vi "DS18S20 - read temp.vi"() -> ()   [LabVIEW 2012]
panel:
  out "Loop Rate (tics)":u32
  in  "stop":bool
  out "Scratchpad Data":u8[](array[numeric]) format="%.0x"
  out "ROM Data":u8[](array[numeric]) format="%.0x"
  out "error out":errorcluster
  in  "error in":errorcluster
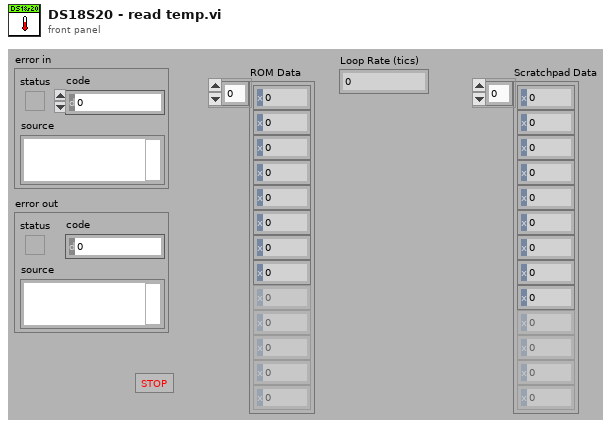
[diagram p1: front panel]
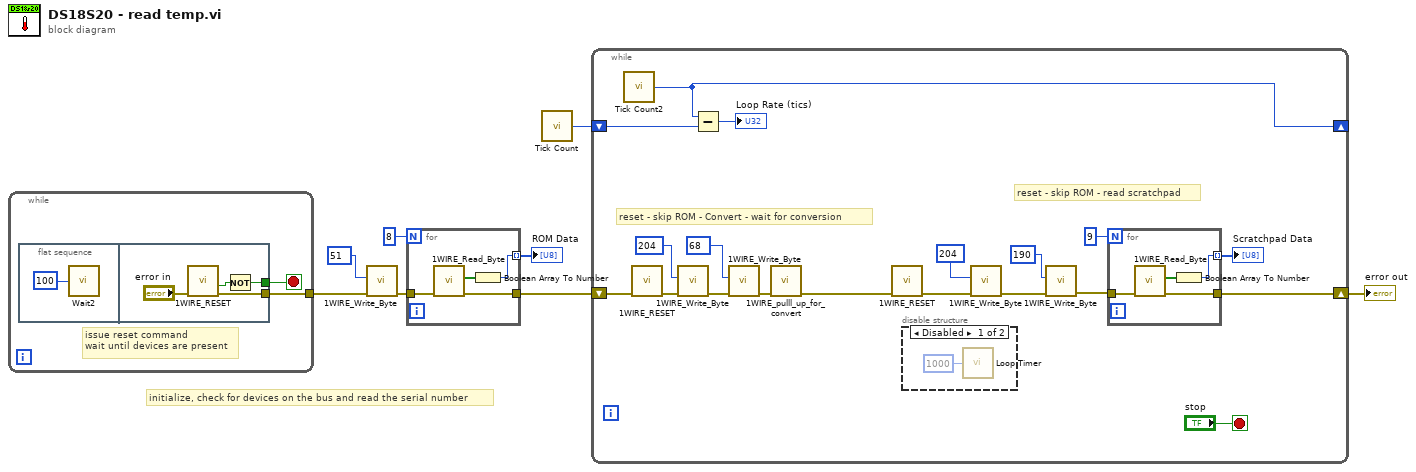
[diagram p0: block diagram]
diagram:
  # "initialize, check for devices on the bus and read the serial number"
  n1 = while {
    tunnel: [w9] -> w4
    stop <- w10 stop-if-true
    # "issue reset command\nwait until devices are present"
    n2 = flat-sequence {
      tunnel: [w15] -> w10
      tunnel: [w14] -> w9
      frame #0 {
        n3 = call "Wait2"("Count(mSec)"=u32 100) -> ()  [unwired: 1 out]
      }
      frame #1 {
        n4 = call "1WIRE_RESET.vi"("error in"="error in") -> ("error out"=w14:errorcluster, "0 = Device Present / 1=no"=w12:bool)  [unwired: 9 in]
        n5 = Not(x=w12) -> (.not. x?=w15:bool)
      }
    }
  }
  n6 = call "1WIRE_Write_Byte.vi"("error in"=w4, "Tx data"=u8 51 ("Tx data 2")) -> ("error out"=w6:errorcluster)  [unwired: 8 in, 1 out]
  n7 = for {
    N: 8 -> [_]
    tunnel: w6 -> [w19]
    tunnel: [w18] -> w1
    tunnel: [w16] -> w8 mode=indexing
    n8 = call "1WIRE_Read_Byte.vi"("error in"=w19) -> ("error out"=w18:errorcluster, "Array"=w17:bool[])  [unwired: 9 in]
    n9 = Boolean Array To Number(Boolean array=w17) -> (number=w16:u8)
  }
  "ROM Data" <- w8
  n10 = call "Tick Count"() -> ("Tick Count(Ticks)"=w3:u32)
  n11 = while {
    shift-right: [w29] -> _
    shift-left: w3 -> [w30]
    shift-right: [w20] -> w2
    shift-left: w1 -> [w27]
    stop <- "stop" stop-if-true
    # "reset - skip ROM - read scratchpad"
    # "reset - skip ROM - Convert - wait for conversion"
    n12 = call "Tick Count2"() -> ("Tick Count(Ticks)"=w29:u32)
    n13 = call "1WIRE_RESET.vi"("error in"=w27) -> ("error out"=w23:errorcluster)  [unwired: 9 in, 1 out]
    n14 = call "1WIRE_Write_Byte.vi"("error in"=w23, "Tx data"=u8 204) -> ("error out"=w22:errorcluster)  [unwired: 8 in, 1 out]
    n15 = Subtract(x=w29, y=w30) -> (x-y=→"Loop Rate (tics)":u32)
    n16 = call "1WIRE_Write_Byte.vi"("error in"=w22, "Tx data"=u8 68 ("Tx data 2")) -> ("error out"=w24:errorcluster)  [unwired: 8 in, 1 out]
    n17 = call "1WIRE_pulll_up_for_convert.vi"("error in"=w24) -> ("error out"=w21:errorcluster)  [unwired: 10 in]
    n18 = call "1WIRE_RESET.vi"("error in"=w21) -> ("error out"=w32:errorcluster)  [unwired: 9 in, 1 out]
    n19 = disable-structure shown="Disabled" {
      frame Disabled {
        n20 = call "Loop Timer"("Count(mSec)"=u32 1000) -> ()  [unwired: 1 out]
      }
      frame Enabled {
      }
    }
    n21 = call "1WIRE_Write_Byte.vi"("error in"=w32, "Tx data"=u8 204) -> ("error out"=w31:errorcluster)  [unwired: 8 in, 1 out]
    n22 = call "1WIRE_Write_Byte.vi"("error in"=w31, "Tx data"=u8 190 ("Tx data 2")) -> ("error out"=w37:errorcluster)  [unwired: 8 in, 1 out]
    n23 = for {
      N: 9 -> [_]
      tunnel: w37 -> [w43]
      tunnel: [w42] -> w20
      tunnel: [w40] -> w35 mode=indexing
      n24 = call "1WIRE_Read_Byte.vi"("error in"=w43) -> ("error out"=w42:errorcluster, "Array"=w41:bool[])  [unwired: 9 in]
      n25 = Boolean Array To Number(Boolean array=w41) -> (number=w40:u8)
    }
    "Scratchpad Data" <- w35
  }
  "error out" <- w2
